vi "WriteObsInfo.vi"(4 "error in (no error)":errorcluster, 5 "# of Entries (before)":i16, 6 "Obs parameters":T1, 7 "Path to FITS Header File":path) -> (0 "error out":errorcluster, 2 "# of Entries (after)":i16, 3 "Path to FITS Header File":path)   [LabVIEW 2015]
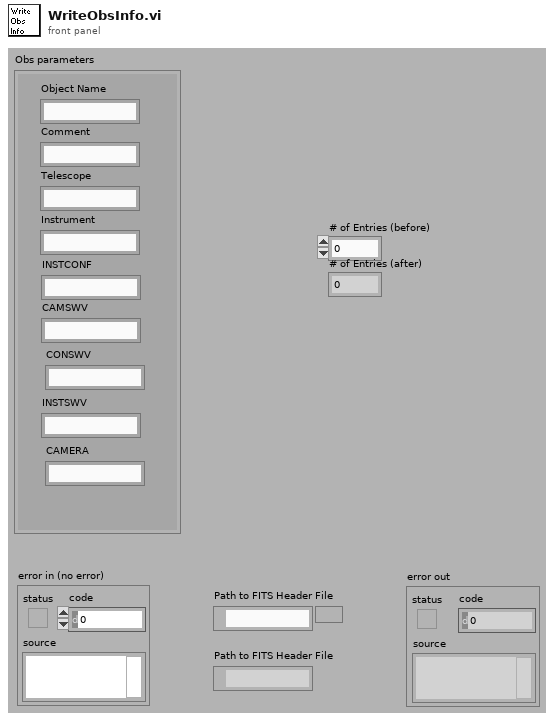
[diagram p1: front panel]
types:
  T1 = cluster{"Object Name":string, "Telescope":string, "Instrument":string, "Comment":string, "INSTCONF":string, "CAMSWV":string, "CONSWV":string, "INSTSWV":string, "CAMERA":string}
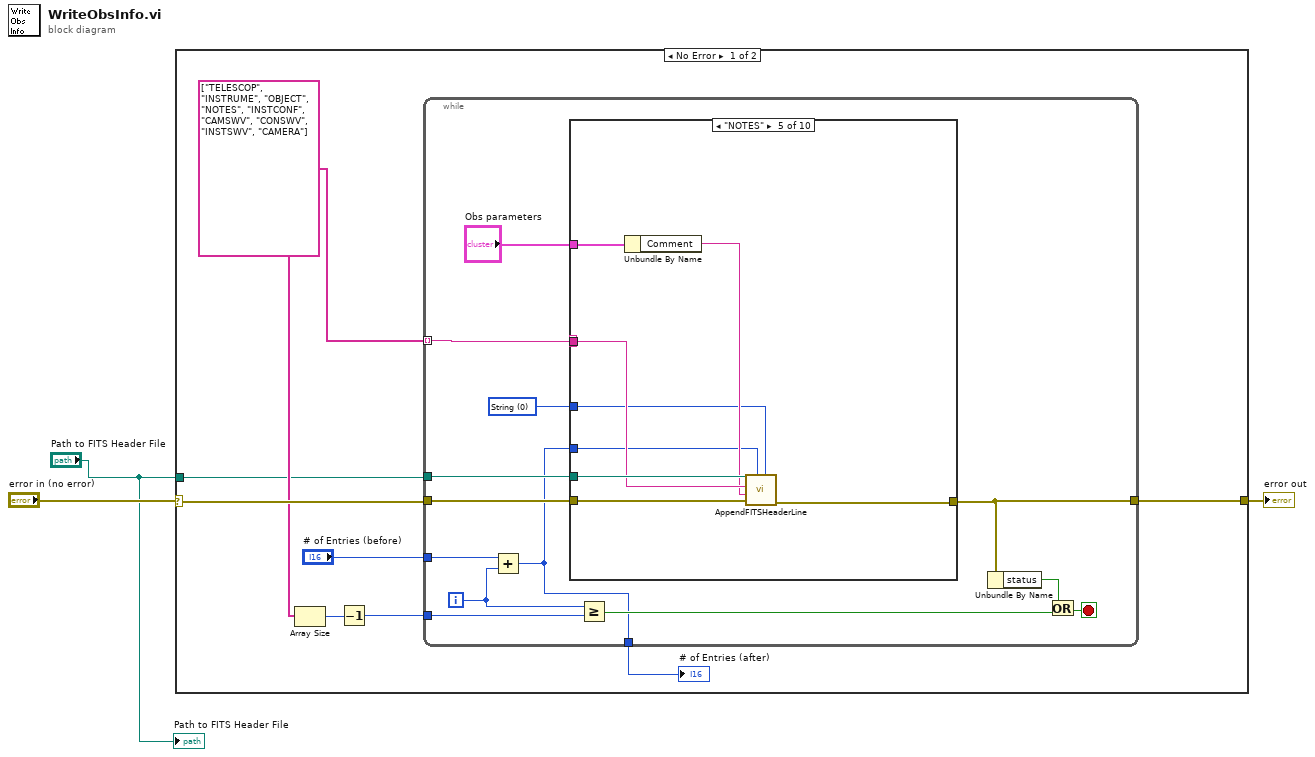
[diagram p0: block diagram]
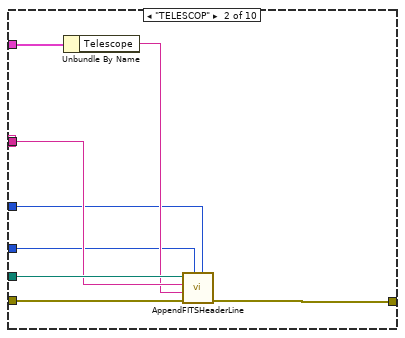
[diagram p3: hidden frame]
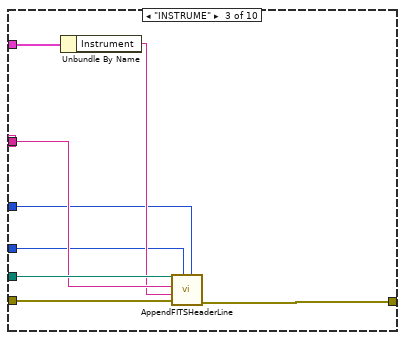
[diagram p4: hidden frame]
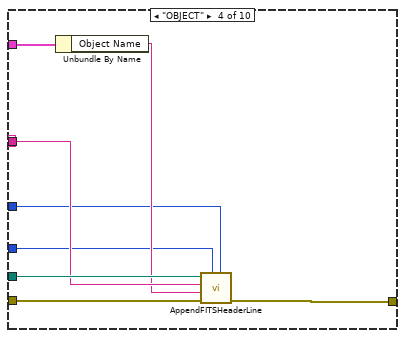
[diagram p5: hidden frame]
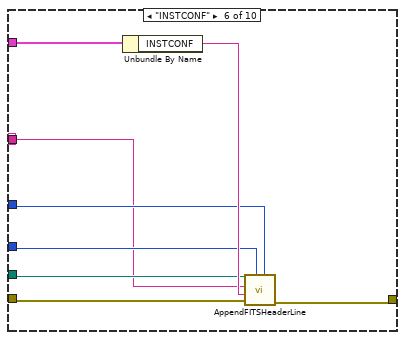
[diagram p6: hidden frame]
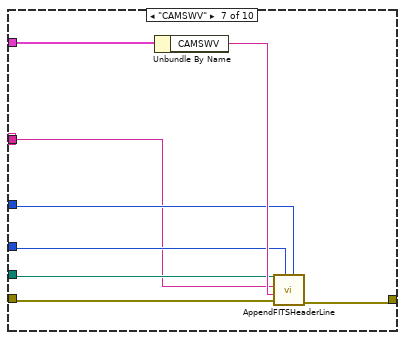
[diagram p7: hidden frame]
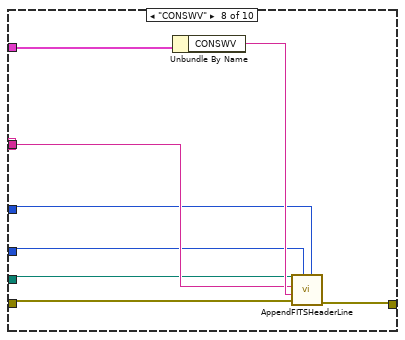
[diagram p8: hidden frame]
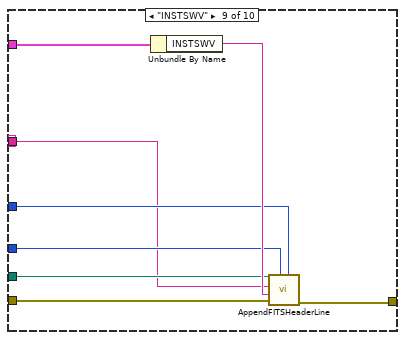
[diagram p9: hidden frame]
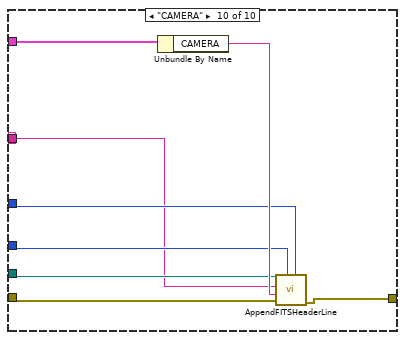
[diagram p10: hidden frame]
diagram:
  n1 = case shown="No Error" "error in (no error)" {
    selector: "error in (no error)" -> [w11 w98]
    tunnel: [w6 w98] -> w3
    tunnel: "Path to FITS Header File" -> [w7 _]
    frame No Error {
      w8 = string[] ["TELESCOP", "INSTRUME", "OBJECT", "NOTES", "INSTCONF", "CAMSWV", "CONSWV", "INSTSWV", "CAMERA"]
      n2 = Array Size(array=w8) -> (size(s)=w10:i32)
      n3 = Decrement(x=w10) -> (x-1=w9:i32)
      n4 = while {
        tunnel: w11 -> [w24]
        tunnel: w8 -> [w17] mode=indexing
        tunnel: w9 -> [w22]
        tunnel: [w21] -> w6
        tunnel: w7 -> [w16]
        tunnel: [w12] -> w5
        tunnel: "# of Entries (before)" -> [w14]
        i -> [w13]
        stop <- w23 stop-if-true
        w15 = u16 0 items=["String", "Numeric", "Boolean"] ("Entry Type")
        n5 = Add(x=w14, y=w13) -> (x+y=w12:i32)
        n6 = case shown="\"NOTES\"" w17 {
          selector: w17 -> [_ w29 w37 w45 w53 w59 w66 w79 w84 w91]
          tunnel: w24 -> [w25 w32 w40 w48 w56 w64 w70 w75 w88 w95]
          tunnel: [w25 w31 w39 w47 w55 w63 w71 w74 w82 w96] -> w21
          tunnel: "Obs parameters" -> [_ w33 w41 w49 w57 w58 w72 w80 w83 w90]
          tunnel: w17 -> [_ _ _ _ _ _ _ _ _ _]
          tunnel: w16 -> [_ w30 w38 w46 w54 w62 w69 w76 w87 w94]
          tunnel: w12 -> [_ w27 w35 w43 w51 w60 w68 w77 w86 w93]
          tunnel: w15 -> [_ w26 w34 w42 w50 w61 w67 w78 w85 w92]
          frame "", Default {
          }
          frame "TELESCOP" {
            n7 = Unbundle By Name(w33) -> ("Telescope"=w28:string)
            n8 = call "AppendFITSHeaderLine.vi"("Entry Type"=w26, "Entry #"=w27, "error in (no error)"=w32, "Element Value"=w28, "Element Name"=w29, "file path (dialog if empty)"=w30) -> ("error out"=w31:errorcluster)  [unwired: 4 in]
          }
          frame "INSTRUME" {
            n9 = Unbundle By Name(w41) -> ("Instrument"=w36:string)
            n10 = call "AppendFITSHeaderLine.vi"("Entry Type"=w34, "Entry #"=w35, "error in (no error)"=w40, "Element Value"=w36, "Element Name"=w37, "file path (dialog if empty)"=w38) -> ("error out"=w39:errorcluster)  [unwired: 4 in]
          }
          frame "OBJECT" {
            n11 = Unbundle By Name(w49) -> ("Object Name"=w44:string)
            n12 = call "AppendFITSHeaderLine.vi"("Entry Type"=w42, "Entry #"=w43, "error in (no error)"=w48, "Element Value"=w44, "Element Name"=w45, "file path (dialog if empty)"=w46) -> ("error out"=w47:errorcluster)  [unwired: 4 in]
          }
          frame "NOTES" {
            n13 = Unbundle By Name(w57) -> ("Comment"=w52:string)
            n14 = call "AppendFITSHeaderLine.vi"("Entry Type"=w50, "Entry #"=w51, "error in (no error)"=w56, "Element Value"=w52, "Element Name"=w53, "file path (dialog if empty)"=w54) -> ("error out"=w55:errorcluster)  [unwired: 4 in]
          }
          frame "INSTCONF" {
            n15 = Unbundle By Name(w58) -> ("INSTCONF"=w65:string)
            n16 = call "AppendFITSHeaderLine.vi"("Entry Type"=w61, "Entry #"=w60, "error in (no error)"=w64, "Element Value"=w65, "Element Name"=w59, "file path (dialog if empty)"=w62) -> ("error out"=w63:errorcluster)  [unwired: 4 in]
          }
          frame "CAMSWV" {
            n17 = Unbundle By Name(w72) -> ("CAMSWV"=w73:string)
            n18 = call "AppendFITSHeaderLine.vi"("Entry Type"=w67, "Entry #"=w68, "error in (no error)"=w70, "Element Value"=w73, "Element Name"=w66, "file path (dialog if empty)"=w69) -> ("error out"=w71:errorcluster)  [unwired: 4 in]
          }
          frame "CONSWV" {
            n19 = Unbundle By Name(w80) -> ("CONSWV"=w81:string)
            n20 = call "AppendFITSHeaderLine.vi"("Entry Type"=w78, "Entry #"=w77, "error in (no error)"=w75, "Element Value"=w81, "Element Name"=w79, "file path (dialog if empty)"=w76) -> ("error out"=w74:errorcluster)  [unwired: 4 in]
          }
          frame "INSTSWV" {
            n21 = Unbundle By Name(w83) -> ("INSTSWV"=w89:string)
            n22 = call "AppendFITSHeaderLine.vi"("Entry Type"=w85, "Entry #"=w86, "error in (no error)"=w88, "Element Value"=w89, "Element Name"=w84, "file path (dialog if empty)"=w87) -> ("error out"=w82:errorcluster)  [unwired: 4 in]
          }
          frame "CAMERA" {
            n23 = Unbundle By Name(w90) -> ("CAMERA"=w97:string)
            n24 = call "AppendFITSHeaderLine.vi"("Entry Type"=w92, "Entry #"=w93, "error in (no error)"=w95, "Element Value"=w97, "Element Name"=w91, "file path (dialog if empty)"=w94) -> ("error out"=w96:errorcluster)  [unwired: 4 in]
          }
        }
        n25 = Greater Or Equal?(x=w13, y=w22) -> (x >= y?=w20:bool)
        n26 = Unbundle By Name(w21) -> ("status"=w19:bool)
        n27 = Or(x=w19, y=w20) -> (x .or. y?=w23:bool)
      }
      "# of Entries (after)" <- w5
    }
    frame Error {
    }
  }
  "error out" <- w3
  "Path to FITS Header File" <- "Path to FITS Header File"
